vi "pyton dpallet car test.vi"(0 "session in":refnum<k35>, 1 "module path 2":path, 2 "function name":string, 3 "Image Src":T1, 4 "img crop":T1, 5 "img out":T1, 6 "image setting cluster in":T2, 7 "error in (no error)":errorcluster) -> (13 "frm false":bool, 14 "return value":dbl[][](array[numeric]), 15 "Image Display":T1(plugin-control), 16 "session out":refnum<k35>, 17 "error out":errorcluster, 18 "Defect Ratio":dbl, 19 "defect type":dbl)   [LabVIEW 2019]
uses:
  <vilib>/vision/Image Controls.llb/IMAQ Image.ctl
  <vilib>/vision/NI_Vision_Development_Module.lvlib
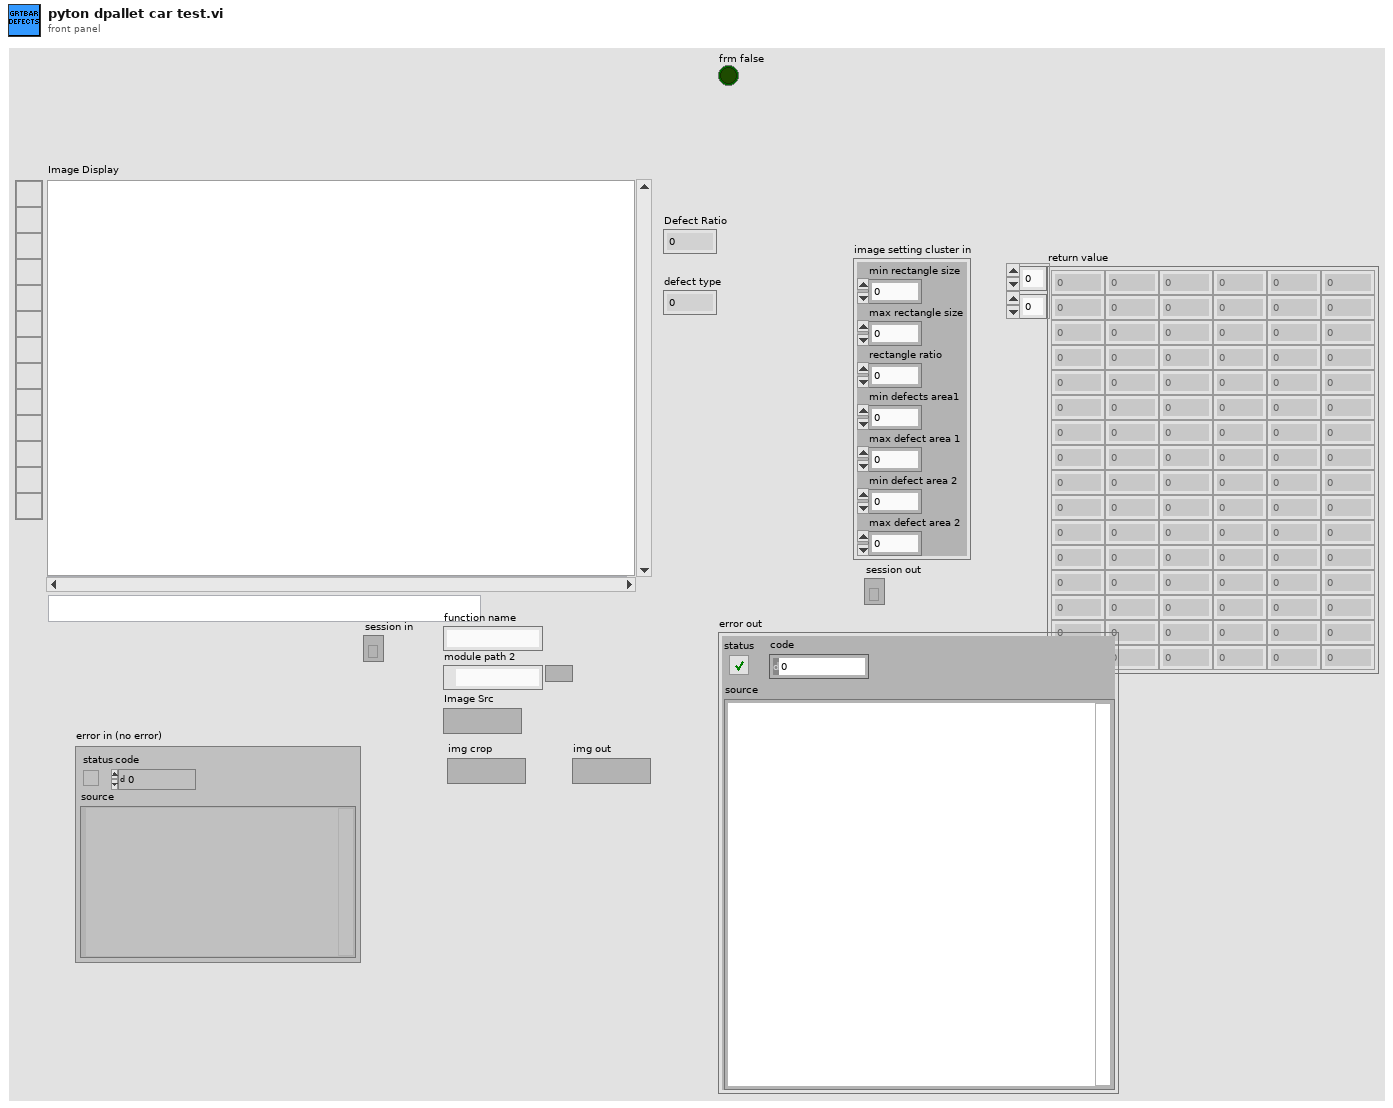
[diagram p1: front panel]
types:
  T1 = typedef "IMAQ Image.ctl" = refnum<image>
  T2 = cluster{"min rectangle size":i32, "max rectangle size":i32, "rectangle ratio":i32, "min defects area1":i32, "max defect area 1":i32, "min defect area 2":i32, "max defect area 2":i32}
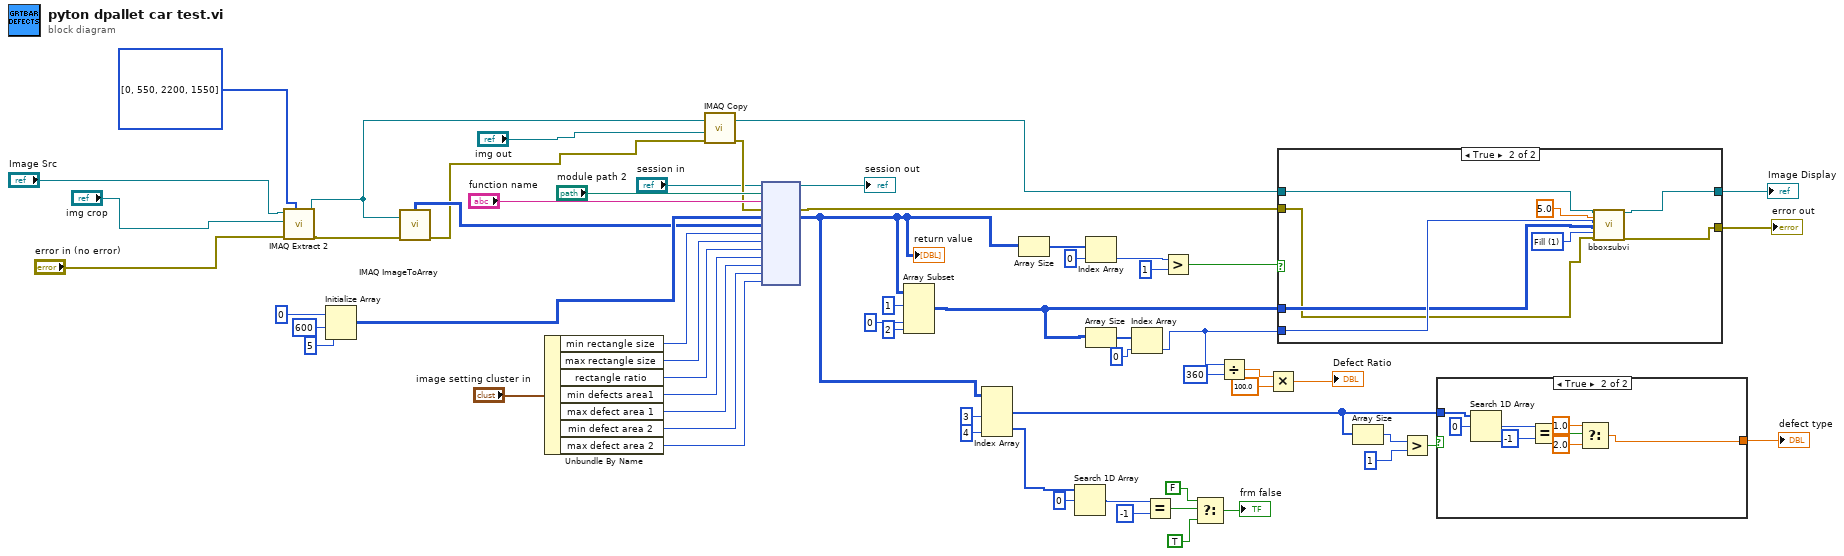
[diagram p0: block diagram]
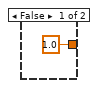
[diagram p2: hidden frame]
diagram:
  n1 = call "IMAQ Extract 2"("Optional Rectangle"=i32[] [0, 550, 2200, 1550], "error in (no error)"="error in (no error)", "Image Dst"="img crop", "Image Src"="Image Src") -> ("error out"=w42:errorcluster, "Image Dst Out"=w43:T1)  [unwired: 6 in]
  n2 = Initialize Array(0 ("element"), 600 ("dimension size"), 5 ("dimension size")) -> (w59:i32[][])
  n3 = call "IMAQ ImageToArray"("error in (no error)"=w42, "Image"=w43) -> ("error out"=w28:errorcluster, "Image Pixels (U8)"=w41:u8[][])  [unwired: 2 in, 3 out]
  n4 = Unbundle By Name("image setting cluster in") -> ("min rectangle size"=w36:i32, "max rectangle size"=w35:i32, "rectangle ratio"=w34:i32, "min defects area1"=w33:i32, "max defect area 1"=w32:i32, "min defect area 2"=w31:i32, "max defect area 2"=w30:i32)
  n5 = call "IMAQ Copy"("error in (no error)"=w28, "Image Dst"="img out", "Image Src"=w43) -> ("error out"=w44:errorcluster, "Image Dst Out"=w48:T1)  [unwired: 3 in]
  n6 = node("session in", "module path 2", "function name", w44, w59, w41, w36, w35, w34, w33, w32, w31, w30) -> (→"session out":refnum<k35>, w47:errorcluster, w9:i32[][])  [unwired: 8 in, 2 out]
  "return value" <- w9
  n7 = Array Subset(array=w9, index (row)=1 ("index"), index (col)=0 ("index"), length (col)=2 ("length")) -> (w16:i32[][])  [unwired: 1 in]
  n8 = Index Array(array=w9, index (col) #1=3 ("disabled index (col)"), index (col) #2=4 ("index (col)")) -> (element #1=w5:i32[], element #2=w6:i32[])  [unwired: 2 in]
  n9 = Array Size(array=w9) -> (size(s)=w53:i32[])
  n10 = Search 1D Array(1D array=w6, element=0) -> (index of element=w13:i32)  [unwired: 1 in]
  n11 = Index Array(array=w53, index=0) -> (element=w51:i32)
  n12 = Array Size(array=w16) -> (size(s)=w24:i32[])
  n13 = Index Array(array=w24, index=0) -> (element=w22:i32)
  n14 = Equal?(x=w13, y=-1) -> (x = y?=w14:bool)
  n15 = Greater?(x=w51, y=1) -> (0:w49:bool)
  n16 = Select(t=FALSE, s=w14, f=TRUE) -> (s? t:f=→"frm false":bool)
  n17 = Divide(x=w22, y=360) -> (x/y=w20:dbl)
  n18 = Multiply(x=w20, y=100.0) -> (x*y=→"Defect Ratio":dbl)
  n19 = case shown="True" w49 {
    tunnel: w48 -> [w64 w72]
    tunnel: w47 -> [w63 w67]
    tunnel: [w64 w66] -> w46
    tunnel: [w63 w65] -> w45
    tunnel: w16 -> [_ w69]
    tunnel: w22 -> [_ w70]
    frame False {
    }
    frame True {
      w68 = u32 1 items=["Frame", "Fill"] ("Drawing Mode (Frame)")
      n20 = call "bboxsubvi.vi"("Image"=w72, "size"=5.0, "def num"=w70, "array"=w69, "Drawing Mode (Frame)"=w68, "error in"=w67) -> ("Image Out"=w66:T1, "error out"=w65:errorcluster)  [unwired: 12 in]
    }
  }
  "error out" <- w45
  "Image Display" <- w46
  n21 = Array Size(array=w5) -> (size(s)=w3:i32)
  n22 = Greater?(x=w3, y=1) -> (0:w4:bool)
  n23 = case shown="True" w4 {
    tunnel: w5 -> [_ w75]
    tunnel: [1.0 ("f") w74] -> w1
    frame False {
    }
    frame True {
      n24 = Search 1D Array(1D array=w75, element=0) -> (index of element=w79:i32)  [unwired: 1 in]
      n25 = Equal?(x=w79, y=-1) -> (x = y?=w80:bool)
      n26 = Select(t=1.0, s=w80, f=2.0) -> (s? t:f=w74:dbl)
    }
  }
  "defect type" <- w1
